vi "App.Open.vi"(8 "error in (no error)":errorcluster, 11 "Cluster":T1) -> (0 "error out":errorcluster)   [LabVIEW 2013, in "Simple Sequence Editor.lvlib"]
uses:
  Simple Sequence Editor.lvlib
  Types/StateVariables.ctl
  Types/ChannelProperties.ctl
  Types/Saved.Sequence.ctl
  Constants.vi
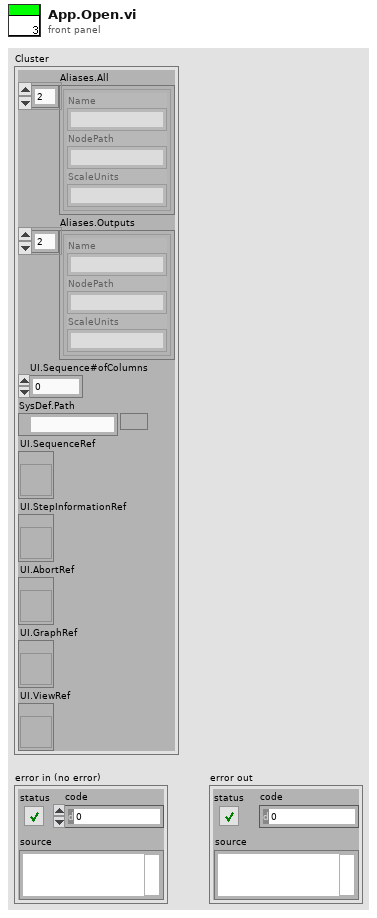
[diagram p1: front panel]
types:
  T1 = typedef "Simple Sequence Editor.lvlib/StateVariables.ctl" = cluster{"Aliases.All":T2[], "Aliases.Outputs":T2[], "UI.Sequence#ofColumns":i32, "SysDef.Path":path, "UI.SequenceRef":refnum<vi>, "UI.StepInformationRef":refnum<vi>, "UI.AbortRef":refnum<vi>, "UI.GraphRef":refnum<vi>, "UI.ViewRef":refnum<vi>}
  T2 = typedef "Simple Sequence Editor.lvlib/ChannelProperties.ctl" = cluster{"Name":string, "NodePath":string, "ScaleUnits":string}
  T3 = typedef "Simple Sequence Editor.lvlib/Saved.Sequence.ctl" = cluster{"Output Channels":T2[], "Item Names":string[][], "Step":string, "Abort":string}
  T4 = enum16{"open", "replace", "create", "open or create", "replace or create", "replace or create with confirmation"}
  T5 = typedef "LVBoundsTypeDef.ctl" = cluster{"Width":u32, "Height":u32}
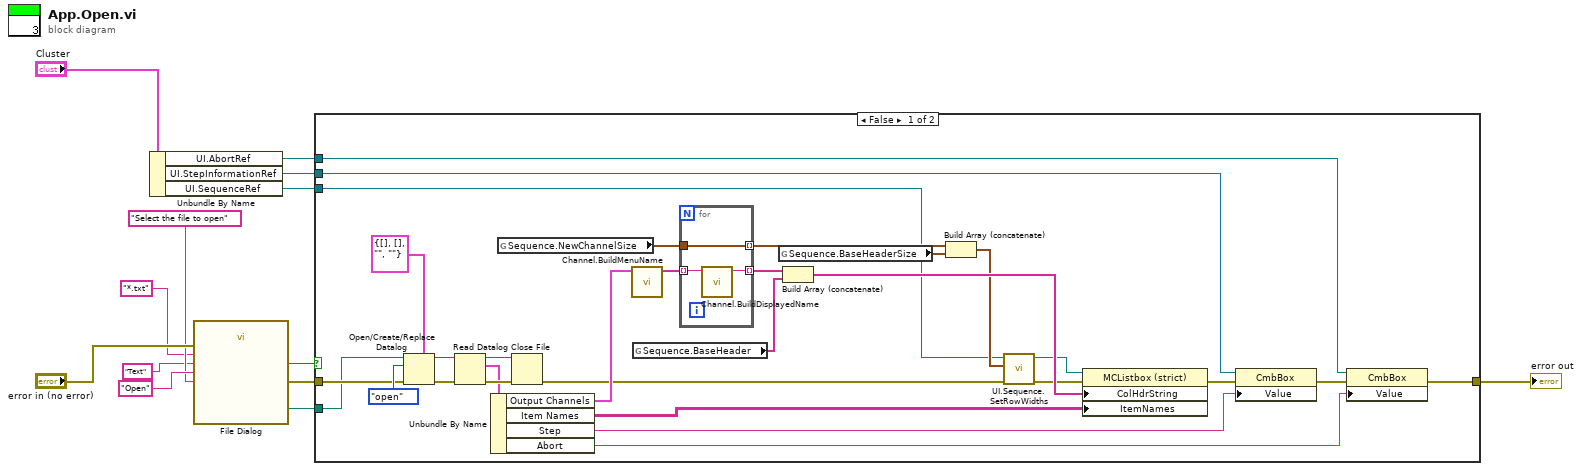
[diagram p0: block diagram]
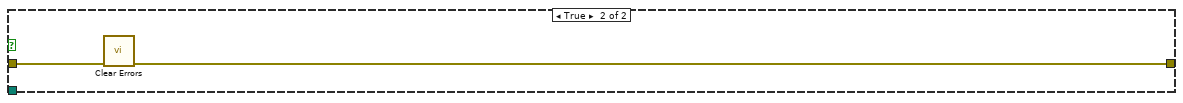
[diagram p2: hidden frame]
diagram:
  n1 = Unbundle By Name("Cluster") -> ("UI.AbortRef"=w13:refnum<vi>, "UI.StepInformationRef"=w12:refnum<vi>, "UI.SequenceRef"=w11:refnum<vi>)
  n2 = call "File Dialog"("prompt"="Select the file to open", "button label"="Open", "error in"="error in (no error)", "pattern (all files)"="*.txt", "pattern label"="Text") -> ("selected path"=w5:path, "cancelled"=w6:bool, "error out"=w1:errorcluster)  [unwired: 7 in, 1 out]
  n3 = case shown="False" w6 {
    tunnel: [w26 w47] -> w9
    tunnel: w1 -> [w38 w48]
    tunnel: w5 -> [w37 _]
    tunnel: w11 -> [w15 _]
    tunnel: w12 -> [w31 _]
    tunnel: w13 -> [w29 _]
    frame False {
      n4 = Open/Create/Replace Datalog(5:T3 {"Output Channels"=[], "Item Names"=[], "Step"="", "Abort"=""}, 8:w38, 10:T4."open" ("operation (0:open)"), 11:w37) -> (0:w43:errorcluster, 3:w40:refnum<k1>)  [unwired: 2 in, 1 out]
      n5 = Read Datalog(4:w43, 7:w40) -> (0:w42:errorcluster, 2:w35:T3, 3:w41:refnum<k1>)  [unwired: 1 in]
      n6 = Unbundle By Name(w35) -> ("Output Channels"=w32:T2[], "Item Names"=w34:string[][], "Step"=w30:string, "Abort"=w28:string)
      n7 = global read "Constants.vi" "Sequence.NewChannelSize"() -> (w22:T5)
      n8 = Close File(refnum=w41, error in=w42) -> (error out=w17:errorcluster)  [unwired: 1 out]
      n9 = call "Channel.BuildMenuName.vi"("Aliases"=w32) -> ("Aliases Array"=w33:string[])  [unwired: 10 in]
      n10 = global read "Constants.vi" "Sequence.BaseHeader"() -> (w23:string[])
      n11 = for {
        tunnel: w33 -> [w46] mode=indexing
        tunnel: [w45] -> w24 mode=indexing
        tunnel: [w44] -> w21 mode=indexing
        tunnel: w22 -> [w44]
        n12 = call "Channel.BuildDisplayedName.vi"("String in"=w46) -> ("String out"=w45:string)  [unwired: 10 in]
      }
      n13 = global read "Constants.vi" "Sequence.BaseHeaderSize"() -> (w20:T5[])
      n14 = Build Array (concatenate)(w24, w23) -> (w25:string[])
      n15 = Build Array (concatenate)(w21, w20) -> (w19:T5[])
      n16 = call "UI.Sequence.SetRowWidths.vi"("error in (no error)"=w17, "Array"=w19, "UI.SequenceRef"=w15) -> ("error out"=w16:errorcluster, "UI.SequenceRef"=w14:refnum<vi>)  [unwired: 7 in]
      n17 = property class="MCListbox (strict)"(reference=w14, error in=w16, "ColHdrString"=w25, "ItemNames"=w34) -> (error out=w18:errorcluster)  [unwired: 1 out]
      n18 = property class="CmbBox"(reference=w31, error in=w18, "Value"=w30) -> (error out=w27:errorcluster)  [unwired: 1 out]
      n19 = property class="CmbBox"(reference=w29, error in=w27, "Value"=w28) -> (error out=w26:errorcluster)  [unwired: 1 out]
    }
    frame True {
      n20 = call <vilib>:"Clear Errors.vi"("error in (no error)"=w48) -> ("error out"=w47:errorcluster)  [unwired: 6 in]
    }
  }
  "error out" <- w9
